vi "CRYSet Limits Front Panel.vi"(11 "Vi Ref":refnum<vi>) -> ()   [LabVIEW 2013]
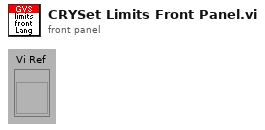
[diagram p1: front panel]
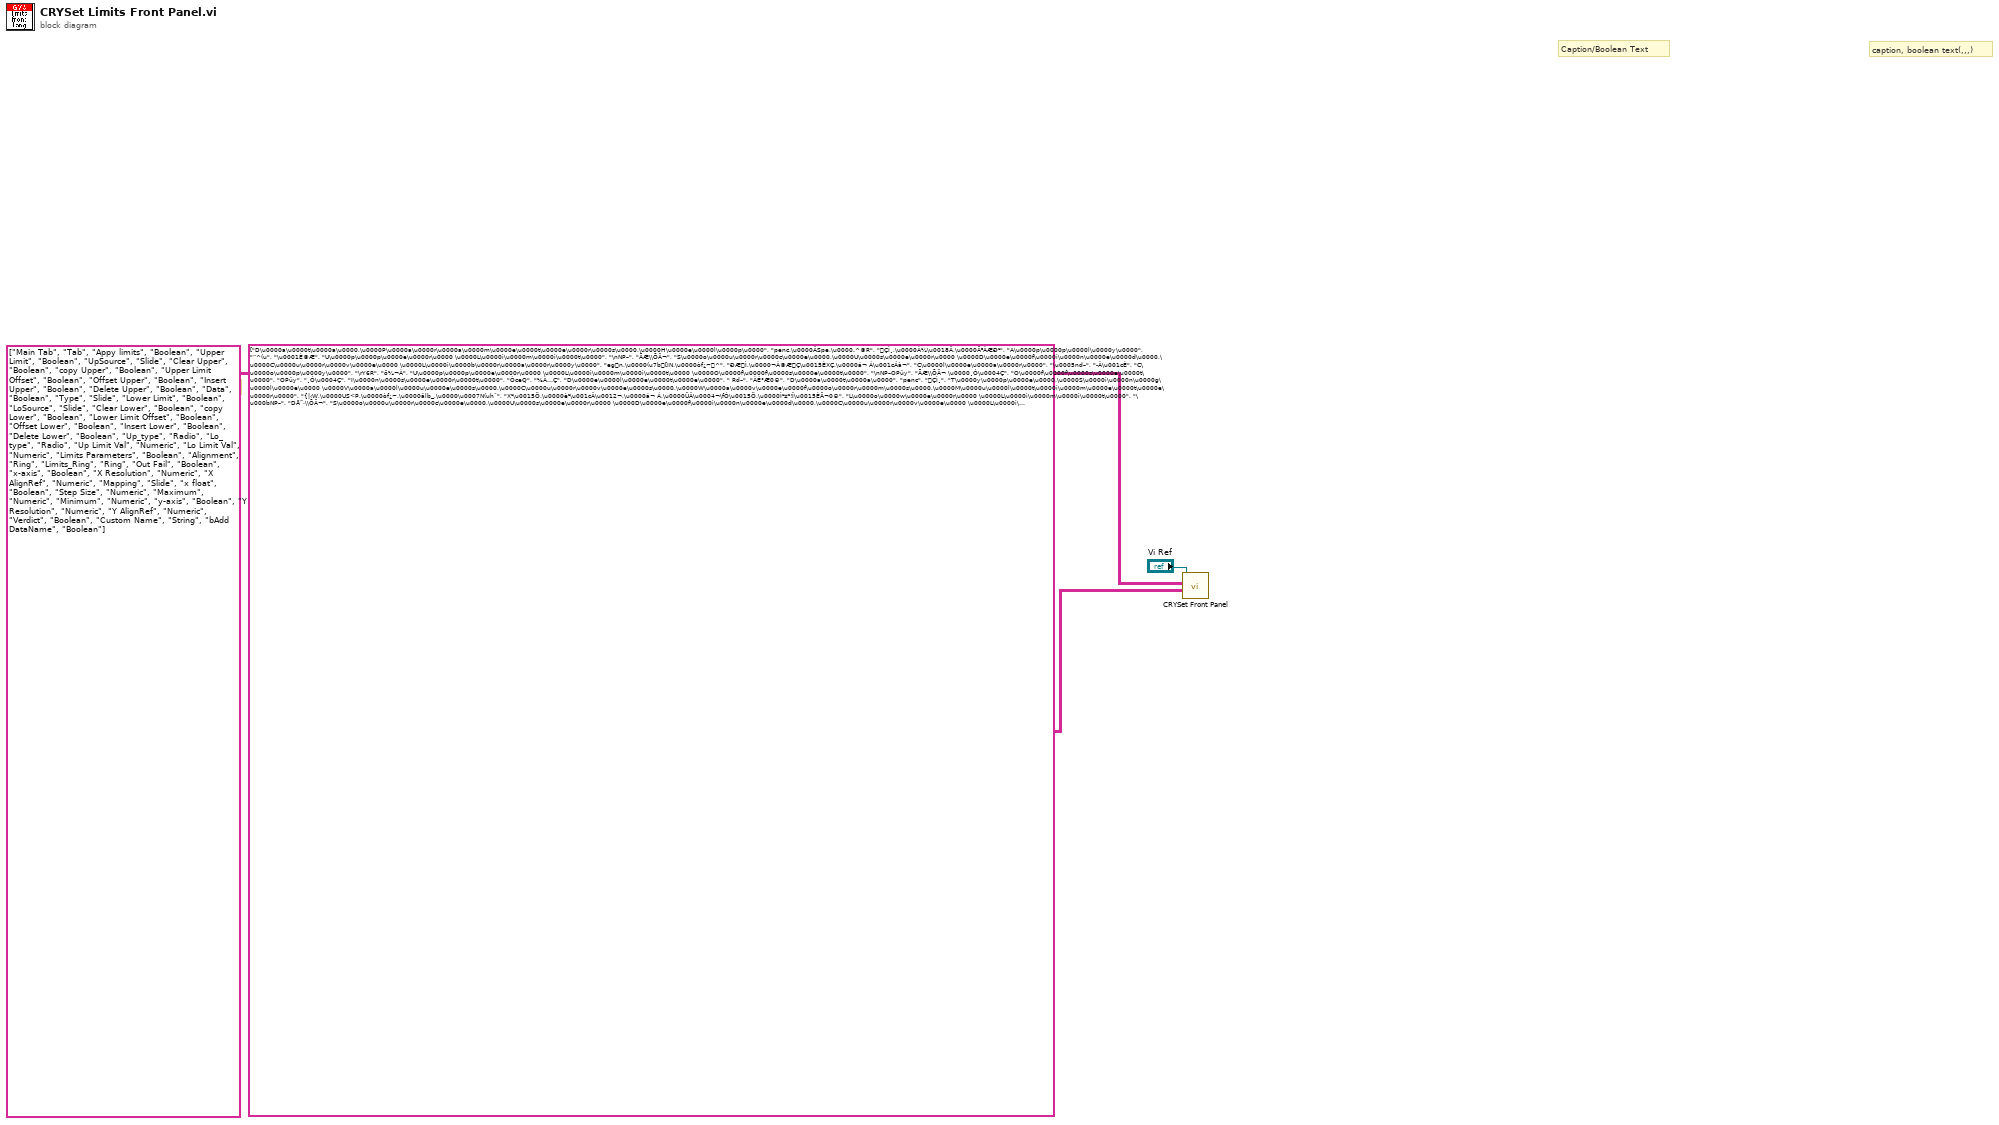
[diagram p0: block diagram]
diagram:
  # "Caption, Tab Page, Multilist Header, Button 4"
  # "Control Type"
  # "Control Name and Tab"
  # "caption, boolean text(,,,)"
  # "Caption/Boolean Text"
  n1 = call "CRYSet Front Panel.vi"("Caption(Boolean Text)"=string[][] [["D\u0000a\u0000t\u0000a\u0000,\u0000P\u0000a\u0000r\u0000a\u0000m\u0000e\u0000t\u0000e\u0000r\u0000s\u0000,\u0000H\u0000e\u0000l\u0000p\u0000", "penc,\u0000ÂSpe,\u0000.^©R", "ÇÌ¸,\u0000À¼\u0018Â,\u0000Ä³ÀÆÐ¹"], ["A\u0000p\u0000p\u0000l\u0000y\u0000", "”^(u", "\u0001È©Æ"], ["U\u0000p\u0000p\u0000e\u0000r\u0000 \u0000L\u0000i\u0000m\u0000i\u0000t\u0000", "\nNP–", "ÃÆ\\ÕÄ¬"], ["S\u0000o\u0000u\u0000r\u0000c\u0000e\u0000,\u0000U\u0000s\u0000e\u0000r\u0000 \u0000D\u0000e\u0000f\u0000i\u0000n\u0000e\u0000d\u0000,\u0000C\u0000u\u0000r\u0000v\u0000e\u0000 \u0000L\u0000i\u0000b\u0000r\u0000a\u0000r\u0000y\u0000", "egn,\u0000(u7b[IN,\u0000òf¿~^", "ÐÆÌ,\u0000¬À©ÆÇ\u0015ÈXÇ,\u0000á¬ Á\u001cÁà¬"], ["C\u0000l\u0000e\u0000a\u0000r\u0000", "\u0005nd–", "­À\u001cÈ"], ["C\u0000o\u0000p\u0000y\u0000", "\rY6R", "õ¼¬À"], ["U\u0000p\u0000p\u0000e\u0000r\u0000 \u0000L\u0000i\u0000m\u0000i\u0000t\u0000 \u0000O\u0000f\u0000f\u0000s\u0000e\u0000t\u0000", "\nNP–OPûy", "ÃÆ\\ÕÄ¬ \u0000¸Ó\u0004Ç"], ["O\u0000f\u0000f\u0000s\u0000e\u0000t\u0000", "OPûy", "¸Ó\u0004Ç"], ["I\u0000n\u0000s\u0000e\u0000r\u0000t\u0000", "ÒceQ", "½À…Ç"], ["D\u0000e\u0000l\u0000e\u0000t\u0000e\u0000", " Rd–", "ÀÉ°Æ0®"], ["D\u0000a\u0000t\u0000a\u0000", "penc", "ÇÌ¸"], ["T\u0000y\u0000p\u0000e\u0000,\u0000S\u0000i\u0000n\u0000g\u0000l\u0000e\u0000 \u0000V\u0000a\u0000l\u0000u\u0000e\u0000s\u0000,\u0000C\u0000u\u0000r\u0000v\u0000e\u0000s\u0000,\u0000W\u0000a\u0000v\u0000e\u0000f\u0000o\u0000r\u0000m\u0000s\u0000,\u0000M\u0000u\u0000l\u0000t\u0000i\u0000m\u0000e\u0000t\u0000e\u0000r\u0000", "{|‹W,\u0000US<P,\u0000òf¿~,\u0000âlb_,\u0000\u0007N(uhˆ", "X¹\u0015Ö,\u0000è²\u001cÂ\u0012¬,\u0000á¬ Á,\u0000ÜÂ\u0004¬\fÓ\u0015Ö,\u0000Ì¹¥²!Î\u0015ÈÄ¬0®"], ["L\u0000o\u0000w\u0000e\u0000r\u0000 \u0000L\u0000i\u0000m\u0000i\u0000t\u0000", "\u000bNP–", "DÅ˜·\\ÕÄ¬"], ["S\u0000o\u0000u\u0000r\u0000c\u0000e\u0000,\u0000U\u0000s\u0000e\u0000r\u0000 \u0000D\u0000e\u0000f\u0000i\u0000n\u0000e\u0000d\u0000,\u0000C\u0000u\u0000r\u0000v\u0000e\u0000 \u0000L\u0000i\u0000b\u0000r\u0000a\u0000r\u0000y\u0000", "egn,\u0000(u7b[IN,\u0000òf¿~^", "ÐÆÌ,\u0000¬À©ÆÇ\u0015ÈXÇ,\u0000á¬ Á\u001cÁà¬"], ["C\u0000l\u0000e\u0000a\u0000r\u0000", "\u0005nd–", "­À\u001cÈ"], ["C\u0000o\u0000p\u0000y\u0000", "\rY6R", "õ¼¬À"], ["L\u0000o\u0000w\u0000e\u0000r\u0000 \u0000L\u0000i\u0000m\u0000i\u0000t\u0000 \u0000O\u0000f\u0000f\u0000s\u0000e\u0000t\u0000", "\u000bNP–OPûy", "DÅ˜·\\ÕÄ¬ \u0000¸Ó\u0004Ç"], ["O\u0000f\u0000f\u0000s\u0000e\u0000t\u0000", "OPûy", "¸Ó\u0004Ç"], ["I\u0000n\u0000s\u0000e\u0000r\u0000t\u0000", "ÒceQ", "½À…Ç"], ["D\u0000e\u0000l\u0000e\u0000t\u0000e\u0000", " Rd–", "ÀÉ°Æ0®"], ["T\u0000y\u0000p\u0000e\u0000,\u0000S\u0000i\u0000n\u0000g\u0000l\u0000e\u0000 \u0000V\u0000a\u0000l\u0000u\u0000e\u0000s\u0000,\u0000C\u0000u\u0000r\u0000v\u0000e\u0000s\u0000,\u0000W\u0000a\u0000v\u0000e\u0000f\u0000o\u0000r\u0000m\u0000s\u0000", "{|‹W,\u0000US<P,\u0000òf¿~,\u0000âlb_", "X¹\u0015Ö,\u0000\u0010È,\u0000á¬ Á,\u0000\fÓ\u0015Ö"], ["T\u0000y\u0000p\u0000e\u0000,\u0000S\u0000i\u0000n\u0000g\u0000l\u0000e\u0000 \u0000V\u0000a\u0000l\u0000u\u0000e\u0000s\u0000,\u0000C\u0000u\u0000r\u0000v\u0000e\u0000s\u0000,\u0000W\u0000a\u0000v\u0000e\u0000f\u0000o\u0000r\u0000m\u0000s\u0000", "{|‹W,\u0000US<P,\u0000òf¿~,\u0000âlb_", "X¹\u0015Ö,\u0000\u0010È,\u0000á¬ Á,\u0000\fÓ\u0015Ö"], ["U\u0000p\u0000p\u0000e\u0000r\u0000 \u0000L\u0000i\u0000m\u0000i\u0000t\u0000", "\nNP–", "ÃÆ\\ÕÄ¬"], ["L\u0000o\u0000w\u0000e\u0000r\u0000 \u0000L\u0000i\u0000m\u0000i\u0000t\u0000", "\u000bNP–", "DÅ˜·\\ÕÄ¬"], ["L\u0000i\u0000m\u0000i\u0000t\u0000s\u0000 \u0000P\u0000a\u0000r\u0000a\u0000m\u0000e\u0000t\u0000e\u0000r\u0000s\u0000", "\nN\u000bNP–ÂSpe", "ù­\\Õ\fÓ|·Tº0Ñ"], ["A\u0000l\u0000i\u0000g\u0000n\u0000m\u0000e\u0000n\u0000t\u0000,\u0000I\u0000n\u0000d\u0000i\u0000v\u0000i\u0000d\u0000u\u0000a\u0000l\u0000 \u0000P\u0000o\u0000i\u0000n\u0000t\u0000s\u0000,\u0000A\u0000b\u0000s\u0000o\u0000l\u0000u\u0000t\u0000e\u0000 \u0000L\u0000i\u0000m\u0000i\u0000t\u0000s\u0000,\u0000F\u0000l\u0000o\u0000a\u0000t\u0000i\u0000n\u0000g\u0000 \u0000L\u0000i\u0000m\u0000i\u0000t\u0000s\u0000,\u0000F\u0000l\u0000o\u0000a\u0000t\u0000i\u0000n\u0000g\u0000 \u0000D\u0000a\u0000t\u0000a\u0000,\u0000A\u0000l\u0000i\u0000g\u0000n\u0000e\u0000d\u0000 \u0000L\u0000i\u0000m\u0000i\u0000t\u0000s\u0000,\u0000A\u0000l\u0000i\u0000g\u0000n\u0000e\u0000d\u0000 \u0000D\u0000a\u0000t\u0000a\u0000", "\nN\u000bNP–ûy¨R¹e\u000f_,\u0000US\u0000N¹p,\u0000Ý~ù[\nN\u000bNP–,\u0000nm¨R\nN\u000bNP–,\u0000nm¨Rpenc,\u0000s^ûy\nN\u000bNP–,\u0000\u0003Œtepenc", "\u0011ÉìÂpÈ\u0015È,\u0000\u001c¬Ä¼\u0001ÈxÇ \u0000\u0010Èä´,\u0000\bÈ\u0000³\u0001ÈxÇ \u0000\\ÕÄ¬,\u0000X¹Ù³XÕ² \u0000\\ÕÄ¬,\u0000X¹Ù³XÕ² \u0000ÇÌ¸,\u0000\u0015È,¸\u001c´ \u0000\\ÕÄ¬,\u0000\u0015È,¸\u001c´ \u0000ÇÌ¸"], ["L\u0000i\u0000m\u0000i\u0000t\u0000s\u0000,\u0000U\u0000p\u0000p\u0000e\u0000r\u0000 \u0000O\u0000n\u0000l\u0000y\u0000,\u0000L\u0000o\u0000w\u0000e\u0000r\u0000 \u0000O\u0000n\u0000l\u0000y\u0000,\u0000U\u0000p\u0000p\u0000e\u0000r\u0000 \u0000&\u0000 \u0000L\u0000o\u0000w\u0000e\u0000r\u0000", "\nN\u000bNP–{|‹W,\u0000êS\tg\nNP–,\u0000êS\tg\u000bNP–,\u0000\nNP–ŒT\u000bNP–", "\\ÕÄ¬,\u0000ÃÆ\\ÕÄ¬,\u0000DÅ˜·\\ÕÄ¬,\u0000ÃÆ\\ÕÄ¬@Æ \u0000DÅ˜·\\ÕÄ¬"], ["O\u0000u\u0000t\u0000p\u0000u\u0000t\u0000 \u0000F\u0000a\u0000i\u0000l\u0000e\u0000d\u0000", "úQ1Y%", "œÍl­äÂ(Ó"], ["x\u0000-\u0000a\u0000x\u0000i\u0000s\u0000", "x\u0000-\u0000t", "x\u0000-\u0000•Í"], ["A\u0000b\u0000s\u0000o\u0000l\u0000u\u0000t\u0000e\u0000 \u0000C\u0000o\u0000m\u0000p\u0000a\u0000r\u0000i\u0000s\u0000o\u0000n\u0000 \u0000P\u0000r\u0000e\u0000c\u0000i\u0000s\u0000i\u0000o\u0000n\u0000", "Ý~ù[Ôk¾|¦^", "\bÈ\u0000³D¾P­\u0015ÈUÖÄ³"], ["A\u0000l\u0000i\u0000g\u0000n\u0000m\u0000e\u0000n\u0000t\u0000 \u0000R\u0000e\u0000f\u0000e\u0000r\u0000e\u0000n\u0000c\u0000e\u0000", "ûy¨RÂS\u0003€¹p", "\u0011ÉìÂ8Ìà¬"], ["M\u0000a\u0000p\u0000p\u0000i\u0000n\u0000g\u0000,\u0000L\u0000i\u0000n\u0000e\u0000a\u0000r\u0000,\u0000L\u0000o\u0000g\u0000", " f\u0004\\,\u0000¿~'`,\u0000ù[pe", "\u0018±0®0®,\u0000 Á\u0015Ö,\u0000\\¸ø­"], ["F\u0000l\u0000o\u0000a\u0000t\u0000 \u0000l\u0000i\u0000m\u0000i\u0000t\u0000s\u0000", "ûy¨RP–6R", "X¹Ù³ù­\\Õ"], ["S\u0000t\u0000e\u0000p\u0000 \u0000S\u0000i\u0000z\u0000e\u0000", "ek¤š'Y\u000f\\", "x¬LÇlÐ0®"], ["M\u0000a\u0000x\u0000i\u0000m\u0000u\u0000m\u0000", "\u0000g'Y", "\\Í\u0000³"], ["M\u0000i\u0000n\u0000i\u0000m\u0000u\u0000m\u0000", "\u0000g\u000f\\", "\\ÍŒÁ"], ["y\u0000-\u0000a\u0000x\u0000i\u0000s\u0000", "y\u0000-\u0000t", "y\u0000-\u0000•Í"], ["A\u0000b\u0000s\u0000o\u0000l\u0000u\u0000t\u0000e\u0000 \u0000C\u0000o\u0000m\u0000p\u0000a\u0000r\u0000i\u0000s\u0000o\u0000n\u0000 \u0000P\u0000r\u0000e\u0000c\u0000i\u0000s\u0000i\u0000o\u0000n\u0000", "Ý~ù[¾|¦^Ôk", "\bÈ\u0000³D¾P­\u0015ÈUÖÄ³"], ["A\u0000l\u0000i\u0000g\u0000n\u0000m\u0000e\u0000n\u0000t\u0000 \u0000R\u0000e\u0000f\u0000e\u0000r\u0000e\u0000n\u0000c\u0000e\u0000", "ûy¨RÂS\u0003€¹p", "\u0011ÉìÂ8Ìà¬"], ["F\u0000a\u0000i\u0000l\u0000e\u0000d\u0000,\u0000P\u0000a\u0000s\u0000s\u0000e\u0000d\u0000", "1Y%,\u0000\u001aÇ", "äÂ(Ó,\u0000µÑü¬"], ["C\u0000u\u0000s\u0000t\u0000o\u0000m\u0000 \u0000R\u0000e\u0000s\u0000u\u0000l\u0000t\u0000 \u0000N\u0000a\u0000m\u0000e\u0000", "ê[IN\rTðy", "¬¹©ÆÇ\u0015ÈXÇ \u0000tÇ¹"], ["A\u0000d\u0000d\u0000 \u0000I\u0000n\u0000p\u0000u\u0000t\u0000 \u0000D\u0000a\u0000t\u0000a\u0000 \u0000N\u0000a\u0000m\u0000e\u0000", " \u0000X ReQpenc\rTðy", "Çl­ÇÌ¸tÇ¹¨Ì½"]], "Control ID and Type(Label Name, Type)"=string[][] [["Main Tab", "Tab"], ["Appy limits", "Boolean"], ["Upper Limit", "Boolean"], ["UpSource", "Slide"], ["Clear Upper", "Boolean"], ["copy Upper", "Boolean"], ["Upper Limit Offset", "Boolean"], ["Offset Upper", "Boolean"], ["Insert Upper", "Boolean"], ["Delete Upper", "Boolean"], ["Data", "Boolean"], ["Type", "Slide"], ["Lower Limit", "Boolean"], ["LoSource", "Slide"], ["Clear Lower", "Boolean"], ["copy Lower", "Boolean"], ["Lower Limit Offset", "Boolean"], ["Offset Lower", "Boolean"], ["Insert Lower", "Boolean"], ["Delete Lower", "Boolean"], ["Up_type", "Radio"], ["Lo_type", "Radio"], ["Up Limit Val", "Numeric"], ["Lo Limit Val", "Numeric"], ["Limits Parameters", "Boolean"], ["Alignment", "Ring"], ["Limits_Ring", "Ring"], ["Out Fail", "Boolean"], ["x-axis", "Boolean"], ["X Resolution", "Numeric"], ["X AlignRef", "Numeric"], ["Mapping", "Slide"], ["x float", "Boolean"], ["Step Size", "Numeric"], ["Maximum", "Numeric"], ["Minimum", "Numeric"], ["y-axis", "Boolean"], ["Y Resolution", "Numeric"], ["Y AlignRef", "Numeric"], ["Verdict", "Boolean"], ["Custom Name", "String"], ["bAdd DataName", "Boolean"]], "Vi Ref"="Vi Ref") -> ()  [unwired: 9 in]
